vi "Close.vi"(8 "error in (no error)":errorcluster, 11 "PXI_MultiTrig in":refnum<class "PXI_MultiTrig.lvclass">) -> (0 "error out":errorcluster, 3 "PXI_MultiTrig out":refnum<class "PXI_MultiTrig.lvclass">)   [LabVIEW 2014, in "SyncPlugins.lvlib" / "PXI_MultiTrig.lvclass"]
uses:
  PXI_MultiTrig.lvclass
  PXI_MultiTrig.lvclass/PXI_MultiTrig.ctl
  SyncPluginBase/SyncPluginBase.lvclass/SyncPluginBase.ctl
  Accessors/Read Clocks.vi
  Accessors/Read Triggers.vi
  Accessors/Read TimingSession.vi
  Accessors/Read RefClkSession.vi
  SyncPluginBase/Accessors/Read Initiated.vi
  Accessors/Write RefClkSession.vi
  Accessors/Write TimingSession.vi
  SyncPluginBase/Accessors/Write Initiated.vi
  SyncPluginBase/Accessors/Write Run.vi
  SyncPluginBase/Accessors/Write Locked.vi
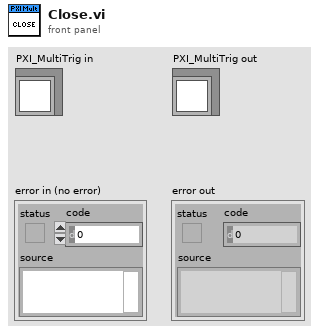
[diagram p1: front panel]
types:
  T1 = typedef "SyncPlugins.lvlib/PXI_MultiTrig.lvclass/clClocks.ctl" = cluster{"Name":string, "RefClk":string, "ClkTerminal":string, "Frequency":dbl, "DutyCycle":dbl, "ClkType":string, "Initiated":bool, "TrigTime":bool}
  T2 = typedef "SyncPlugins.lvlib/PXI_MultiTrig.lvclass/clTrigger.ctl" = cluster{"Name":string, "DestTerm":string, "SrcTerm":string, "SyncClk":string, "Edge":i32, "Invert?":i32, "Initiated":bool, "Type":string, "TrigTime":bool}
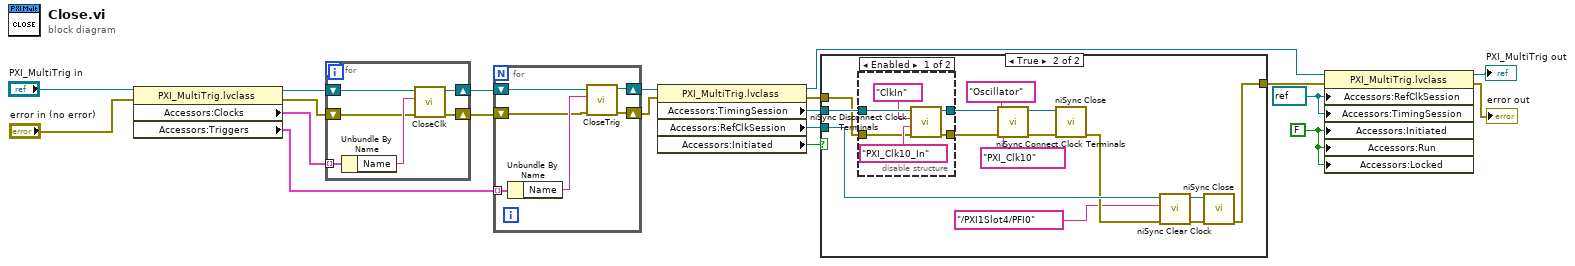
[diagram p0: block diagram]
diagram:
  w5 = refnum<k15> refnum ("RefClkSession")
  w6 = FALSE ("Initiated")
  n1 = property class="PXI_MultiTrig.lvclass"(reference="PXI_MultiTrig in", error in="error in (no error)") -> (reference out=w17:refnum<class "PXI_MultiTrig.lvclass">, error out=w16:errorcluster, "Accessors:Clocks"=w18:T1[], "Accessors:Triggers"=w13:T2[])
  n2 = for {
    tunnel: w18 -> [w26] mode=indexing
    shift-right: [w22] -> w15
    shift-left: w17 -> [w25]
    shift-right: [w21] -> w14
    shift-left: w16 -> [w23]
    n3 = Unbundle By Name(w26) -> ("Name"=w24:string)
    n4 = call-dynamic "CloseClk.vi"("error in (no error)"=w23, "ClkName"=w24, "PXI_MultiTrig in"=w25) -> ("error out"=w21:errorcluster, "PXI_MultiTrig out"=w22:refnum<class "PXI_MultiTrig.lvclass">)  [unwired: 7 in]
  }
  n5 = for {
    shift-right: [w28] -> w12
    shift-left: w15 -> [w27]
    tunnel: w13 -> [w32] mode=indexing
    shift-right: [w29] -> w11
    shift-left: w14 -> [w30]
    n6 = Unbundle By Name(w32) -> ("Name"=w31:string)
    n7 = call-dynamic "CloseTrig.vi"("error in (no error)"=w30, "TrigName"=w31, "PXI_MultiTrig in"=w27) -> ("error out"=w29:errorcluster, "PXI_MultiTrig out"=w28:refnum<class "PXI_MultiTrig.lvclass">)  [unwired: 7 in]
  }
  n8 = property class="PXI_MultiTrig.lvclass"(reference=w12, error in=w11) -> (reference out=w7:refnum<class "PXI_MultiTrig.lvclass">, error out=w9:errorcluster, "Accessors:TimingSession"=w10:refnum<k15>, "Accessors:RefClkSession"=w8:refnum<k15>, "Accessors:Initiated"=w1:bool)
  n9 = case shown="True" w1 {
    tunnel: w10 -> [_ w47]
    tunnel: w9 -> [w33 w46]
    tunnel: w8 -> [_ w38]
    tunnel: [w33 w41] -> w4
    frame False {
    }
    frame True {
      n10 = disable-structure shown="Enabled" {
        disable-tunnel: w47 -> [w53 w55]
        disable-tunnel: w46 -> [w50 w54]
        disable-tunnel: [w49 w54] -> w45
        disable-tunnel: [w48 w55] -> w44
        frame Enabled {
          n11 = call <instrlib>:"niSync Disconnect Clock Terminals.vi"("error in (no error)"=w50, "destination terminal"="PXI_Clk10_In", "source terminal"="ClkIn", "instrument handle"=w53) -> ("error out"=w49:errorcluster, "instrument handle out"=w48:refnum<k15>)  [unwired: 6 in]
        }
        frame Disabled {
        }
      }
      n12 = call <instrlib>:"niSync Connect Clock Terminals.vi"("error in (no error)"=w45, "destination terminal"="PXI_Clk10", "source terminal"="Oscillator", "instrument handle"=w44) -> ("error out"=w43:errorcluster, "instrument handle out"=w42:refnum<k15>)  [unwired: 6 in]
      n13 = call <instrlib>:"niSync Close.vi"("error in (no error)"=w43, "instrument handle"=w42) -> ("error out"=w37:errorcluster)  [unwired: 9 in]
      n14 = call <instrlib>:"niSync Clear Clock.vi"("error in (no error)"=w37, "terminal"=tag "/PXI1Slot4/PFI0", "instrument handle"=w38) -> ("error out"=w35:errorcluster, "instrument handle out"=w34:refnum<k15>)  [unwired: 6 in]
      n15 = call <instrlib>:"niSync Close.vi"("error in (no error)"=w35, "instrument handle"=w34) -> ("error out"=w41:errorcluster)  [unwired: 9 in]
    }
  }
  n16 = property class="PXI_MultiTrig.lvclass"(reference=w7, error in=w4, "Accessors:RefClkSession"=w5, "Accessors:TimingSession"=w5, "Accessors:Initiated"=w6, "Accessors:Run"=w6, "Accessors:Locked"=w6) -> (reference out=→"PXI_MultiTrig out":refnum<class "PXI_MultiTrig.lvclass">, error out=→"error out":errorcluster)
